vi "Read_Data.vi"(8 "error in":errorcluster) -> (0 "error out":errorcluster, 3 "string array":string[](array[string]))   [LabVIEW 2021]
panel:
  out "standard error":string
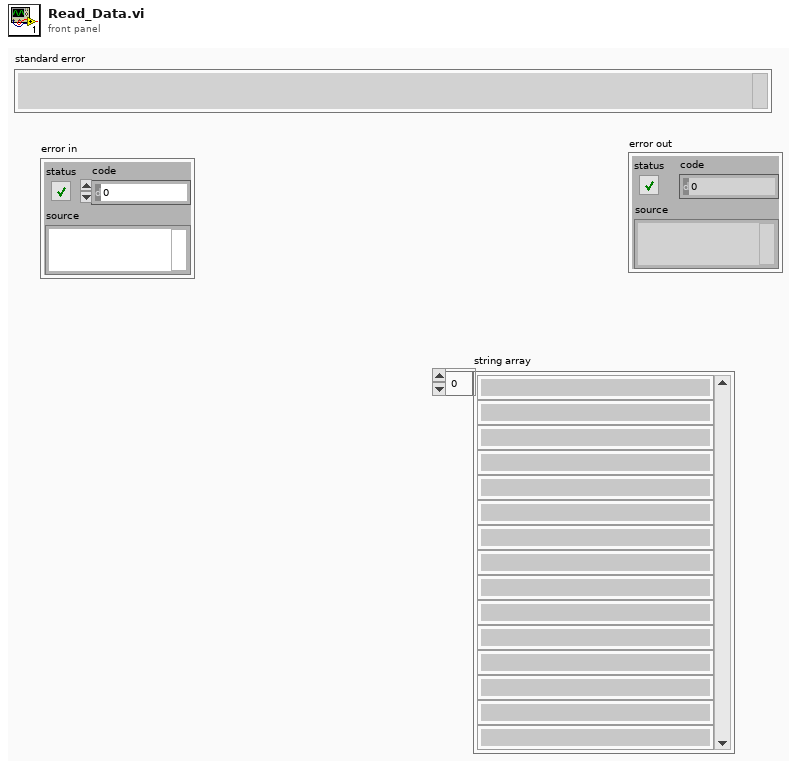
[diagram p1: front panel]
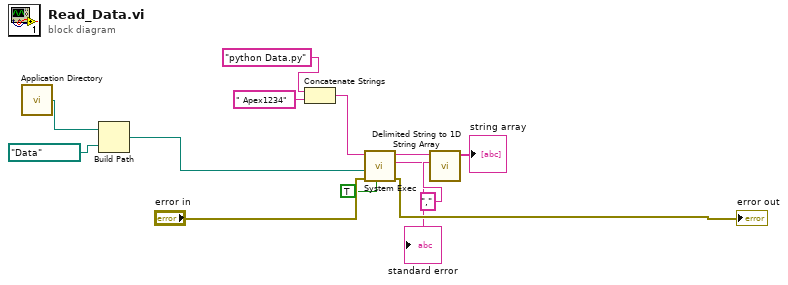
[diagram p0: block diagram]
diagram:
  n1 = call <vilib>:"Application Directory.vi"() -> ("Application Directory"=w4:path)
  n2 = Build Path(base path=w4, name or relative path=path "Data" ("working directory")) -> (appended path=w2:path)
  n3 = Concatenate Strings("python Data.py" ("command line"), " Apex1234" ("string")) -> (w8:string)
  n4 = call <vilib>:"System Exec.vi"("run minimized? (F)"=TRUE, "error in (no error)"="error in", "working directory"=w2, "command line"=w8) -> ("error out"=→"error out":errorcluster, "standard error"=→"standard error":string, "standard output"=w11:string)  [unwired: 4 in, 1 out]
  n5 = call <vilib>:"Delimited String to 1D String Array.vi"("delimiter"=",", "delimited string"=w11) -> ("string array"=→"string array":string[])  [unwired: 9 in]
